vi "get supported measurement types.vi"(8 "error in":errorcluster, 11 "Daqmx Module configuration in":refnum<class "DAQmx Module Configuration.lvclass">) -> (0 "error out":errorcluster, 2 "supported measurement  types":T1[](array[typedef])=[enum."Digital Input", enum."Digital Output", enum."Voltage Input", enum."Voltage Output", enum."Current Input", enum."Current Output", enum."RTD", enum."Thermocouple", enum."Strain"], 3 "Daqmx Module configuration out":refnum<class "DAQmx Module Configuration.lvclass">)   [LabVIEW 2014, in "DAQmx Module Configuration.lvclass"]
doc: "Provides an interface for determining the targets supported by a given configuration/runtime class pairing. This should be overridden by any useful child class."
uses:
  DAQmx Module Configuration.lvclass
  Measurement Type.ctl
  <vilib>/NI/Tag Bus/tag/tag descriptor.lvclass
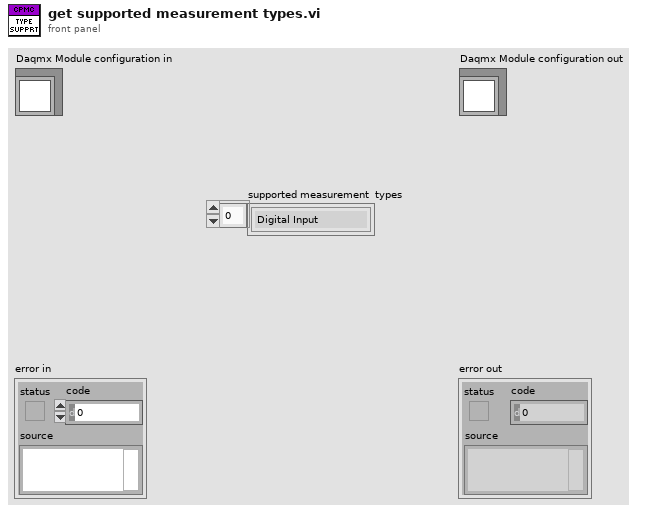
[diagram p1: front panel]
types:
  T1 = typedef "DAQmx Module Configuration.lvclass/Measurement Type.ctl" = enum16{"Digital Input", "Digital Output", "Voltage Input", "Voltage Output", "Current Input", "Current Output", "RTD", "Thermocouple", "Strain"}
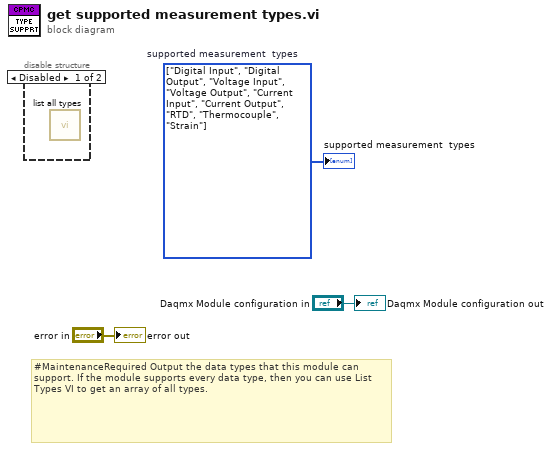
[diagram p0: block diagram]
diagram:
  w1 = T1[] [enum."Digital Input", enum."Digital Output", enum."Voltage Input", enum."Voltage Output", enum."Current Input", enum."Current Output", enum."RTD", enum."Thermocouple", enum."Strain"] items=["Digital Input", "Digital Output", "Voltage Input", "Voltage Output", "Current Input", "Current Output", "RTD", "Thermocouple", "Strain"]  # supported measurement  types
  # "#MaintenanceRequired Output the data types that this module can support. If the module supports every data type, then you can use List Types VI to get an array of all types."
  n1 = disable-structure shown="Disabled" {
    frame Disabled {
      n2 = call <vilib>:"list all types.vi"() -> ()  [unwired: 11 in, 1 out]
    }
    frame Enabled {
    }
  }
  "error out" <- "error in"
  "Daqmx Module configuration out" <- "Daqmx Module configuration in"
  "supported measurement  types" <- w1
